vi "Clear INI Settings.vi"(10 "Variant":variant) -> (0 "error out":errorcluster)   [LabVIEW 2020]
uses:
  Toolbox/LMH-Toolbox.lvlib
  <vilib>/zip/NI_Unzip.lvlib
panel:
  out "LinxProviderError":errorcluster
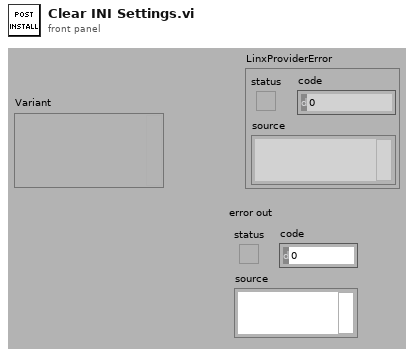
[diagram p1: front panel]
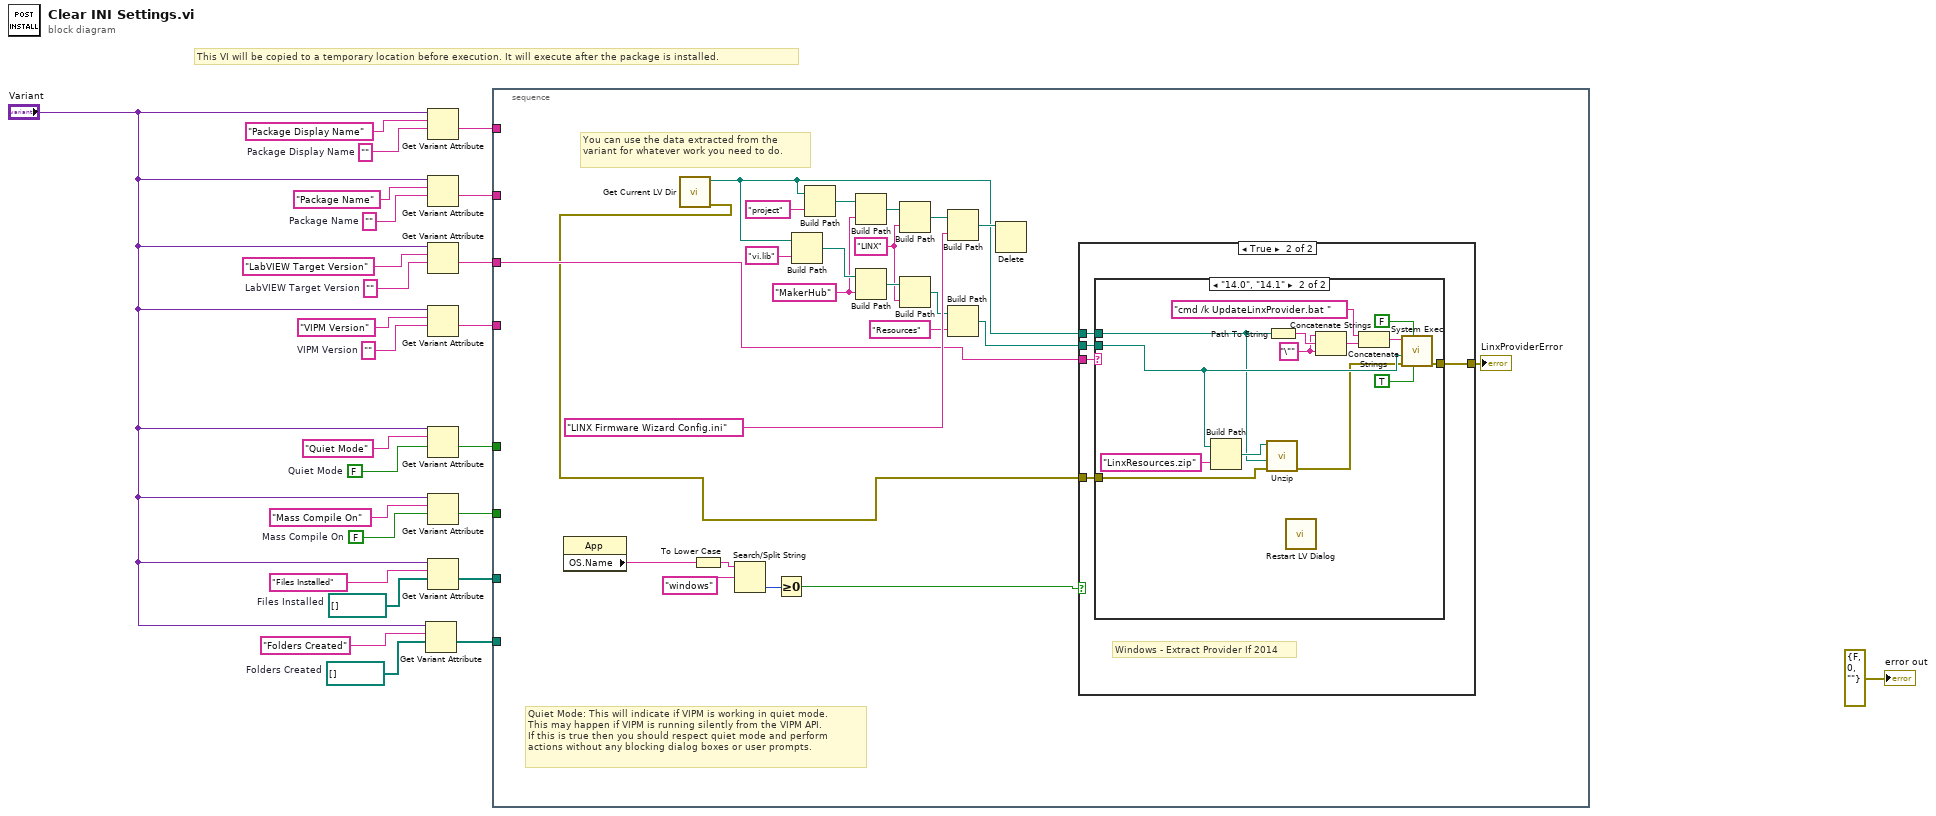
[diagram p0: block diagram]
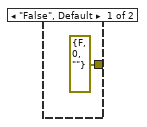
[diagram p3: hidden frame]
diagram:
  w1 = path[] []  # Folders Created
  w2 = path[] []  # Files Installed
  w8 = FALSE  # Mass Compile On
  w9 = ""  # Package Display Name
  w16 = FALSE  # Quiet Mode
  w19 = ""  # VIPM Version
  w21 = ""  # LabVIEW Target Version
  w23 = ""  # Package Name
  # "This VI will be copied to a temporary location before execution. It will execute after the package is installed."
  n1 = Get Variant Attribute(Variant="Variant", name="Folders Created", default value (empty Variant)=w1) -> (value=w6:path[])  [unwired: 1 in, 3 out]
  n2 = Get Variant Attribute(Variant="Variant", name="Package Display Name", default value (empty Variant)=w9) -> (value=w15:string)  [unwired: 1 in, 3 out]
  n3 = Get Variant Attribute(Variant="Variant", name="Package Name", default value (empty Variant)=w23) -> (value=w14:string)  [unwired: 1 in, 3 out]
  n4 = Get Variant Attribute(Variant="Variant", name="LabVIEW Target Version", default value (empty Variant)=w21) -> (value=w13:string)  [unwired: 1 in, 3 out]
  n5 = Get Variant Attribute(Variant="Variant", name="VIPM Version", default value (empty Variant)=w19) -> (value=w12:string)  [unwired: 1 in, 3 out]
  n6 = Get Variant Attribute(Variant="Variant", name="Quiet Mode", default value (empty Variant)=w16) -> (value=w11:bool)  [unwired: 1 in, 3 out]
  n7 = Get Variant Attribute(Variant="Variant", name="Mass Compile On", default value (empty Variant)=w8) -> (value=w10:bool)  [unwired: 1 in, 3 out]
  n8 = Get Variant Attribute(Variant="Variant", name="Files Installed", default value (empty Variant)=w2) -> (value=w5:path[])  [unwired: 1 in, 3 out]
  n9 = stacked-sequence {
    tunnel: w15 -> [_]
    tunnel: w14 -> [_]
    tunnel: w13 -> [w38]
    tunnel: w12 -> [_]
    tunnel: w11 -> [_]
    tunnel: w10 -> [_]
    tunnel: w5 -> [_]
    tunnel: w6 -> [_]
    frame #0 {
      w39 = "LINX" ("name or relative path")
      w40 = "MakerHub" ("name or relative path")
      # "Quiet Mode: This will indicate if VIPM is working in quiet mode.\nThis may happen if VIPM is running silently from the VIPM API.\nIf this is true then you should respect quiet mode and perform\nactions without any blocking dialog boxes or user prompts."
      # "You can use the data extracted from the variant for whatever work you need to do."
      n10 = property class="App"() -> ("OS.Name"=w30:string)  [unwired: 2 in, 2 out]
      n11 = call "Get Current LV Dir.vi"() -> ("Error Out"=w32:errorcluster, "This LV Directory"=w34:path)  [unwired: 10 in]
      n12 = To Lower Case(string=w30) -> (all lower case string=w31:string)
      n13 = Search/Split String(string=w31, search string/char (-)="windows") -> (offset of match=w28:i32)  [unwired: 1 in, 2 out]
      n14 = Greater Or Equal To 0?(x=w28) -> (x >= 0?=w27:bool)
      n15 = Build Path(base path=w34, name or relative path="vi.lib") -> (appended path=w42:path)
      n16 = Build Path(base path=w34, name or relative path="project") -> (appended path=w46:path)
      n17 = Build Path(base path=w46, name or relative path=w40) -> (appended path=w45:path)
      n18 = Build Path(base path=w42, name or relative path=w40) -> (appended path=w43:path)
      n19 = Build Path(base path=w45, name or relative path=w39) -> (appended path=w44:path)
      n20 = Build Path(base path=w43, name or relative path=w39) -> (appended path=w33:path)
      n21 = Build Path(base path=w44, name or relative path="LINX Firmware Wizard Config.ini") -> (appended path=w48:path)
      n22 = Build Path(base path=w33, name or relative path="Resources") -> (appended path=w35:path)
      n23 = Delete(path (use dialog)=w48) -> ()  [unwired: 4 in, 3 out]
      n24 = case shown="True" w27 {
        tunnel: w38 -> [_ w55]
        tunnel: [w50 w54] -> w37
        tunnel: w35 -> [_ w53]
        tunnel: w34 -> [_ w52]
        tunnel: w32 -> [w50 w51]
        frame False {
          # "Not Windows.  Don't try to extract LINX Provider"
        }
        frame True {
          # "Windows - Extract Provider If 2014"
          n25 = case shown="\"14.0\", \"14.1\"" w55 {
            tunnel: w53 -> [_ w62]
            tunnel: [errorcluster {"status"=FALSE, "code"=0, "source"=""} ("error out") w63] -> w54
            tunnel: w52 -> [_ w59]
            tunnel: w51 -> [_ w58]
            frame "False", Default {
            }
            frame "14.0", "14.1" {
              w65 = "\"" ("string")
              n26 = Build Path(base path=w62, name or relative path="LinxResources.zip") -> (appended path=w61:path)
              n27 = call <vilib>:"Unzip.vi"("error in (no error)"=w58, "Target directory (same as Zip file if empty)"=w59, "Zip file"=w61) -> ("error out"=w57:errorcluster)  [unwired: 6 in, 2 out]
              n28 = Path To String(path=w59) -> (string=w66:string)
              n29 = call "Restart LV Dialog.vi"() -> ()  [unwired: 12 in]
              n30 = Concatenate Strings(w65, w66, w65) -> (w64:string)
              n31 = Concatenate Strings("cmd /k UpdateLinxProvider.bat " ("command line"), w64) -> (w68:string)
              n32 = call <vilib>:"System Exec.vi"("run minimized? (F)"=TRUE, "wait until completion? (T)"=FALSE, "error in (no error)"=w57, "working directory"=w62, "command line"=w68) -> ("error out"=w63:errorcluster)  [unwired: 3 in, 3 out]
            }
          }
        }
      }
      "LinxProviderError" <- w37
    }
  }
  "error out" <- errorcluster {"status"=FALSE, "code"=0, "source"=""} ("error out")
